vi "Remove Null Characters.vi"(4 "strIn":string) -> (1 "strOut":string)   [LabVIEW 2013]
doc: "This VI is used in conjunction with the Hill Cipher decypt function. If the number of bytes is not a factor of three, then the string will be padded to that number with null bytes. Call this method to remove those null bytes."
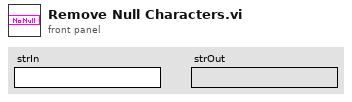
[diagram p1: front panel]
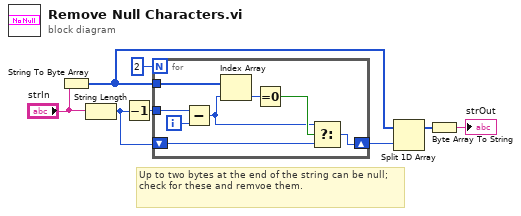
[diagram p0: block diagram]
diagram:
  # "Up to two bytes at the end of the string can be null; check for these and remvoe them."
  n1 = String To Byte Array(string="strIn") -> (unsigned byte array=w5:u8[])
  n2 = String Length(string="strIn") -> (length=w3:i32)
  n3 = Decrement(x=w3) -> (x-1=w2:i32)
  n4 = for {
    N: 2 -> [_]
    tunnel: w5 -> [w14]
    tunnel: w2 -> [w15]
    shift-right: [w9] -> w4
    shift-left: w3 -> [w10]
    i -> [w16]
    n5 = Subtract(x=w15, y=w16) -> (x-y=w11:i32)
    n6 = Index Array(array=w14, index=w11) -> (element=w13:u8)
    n7 = Equal To 0?(x=w13) -> (x = 0?=w12:bool)
    n8 = Select(t=w11, s=w12, f=w10) -> (s? t:f=w9:i32)
  }
  n9 = Split 1D Array(array=w5, index=w4) -> (first subarray=w6:u8[])  [unwired: 1 out]
  n10 = Byte Array To String(unsigned byte array=w6) -> (string=→"strOut":string)
